vi "Teleop.vi"(10 "Match Info":T1={"Autonomous Elapsed Seconds"=0.0, "TeleOp Elapsed Seconds"=0.0, "Disabled Elapsed Seconds"=0.0, "Visited Autonomous"=FALSE, "Visited TeleOp"=FALSE, "Visited Disabled"=FALSE, "Autonomous Settings"={"Autonomous Style"=enum."Independent", "VI Refnum"=refnum}}, 11 "Call Context":T2) -> ()   [LabVIEW 2014]
doc: "This VI is called for each TeleOp packet received from the DS where the robot is not disabled. It is often used to read from the joysticks and update I/O or to update setpoints for timed control loops. It should complete and return within 20 milliseconds or it may miss DS packets."
uses:
  <vilib>/Rock Robotics/WPI/DriverStation/WPI_DriverStationDerivedRobotMode.ctl
  <vilib>/Rock Robotics/WPI/DriverStation/WPI_DriverStationMatch Info.ctl
  <vilib>/Rock Robotics/WPI/Joystick/WPI_JoystickGetSetRefNum.vi
  Robot Global Data.vi
  <vilib>/Rock Robotics/Network Tables/SD Write Boolean Array.vi
  <vilib>/Rock Robotics/Network Tables/SD Write Numeric Array.vi
  <vilib>/Rock Robotics/Network Tables/SD Read Boolean.vi
  <vilib>/Rock Robotics/Network Tables/SD Read Number.vi
  <vilib>/Rock Robotics/WPI/Compressor/WPI_CompressorGetSetRefNum.vi
panel:
  out "Wheel Lock":bool
  out "Closed Loop":bool
  out "Record":bool
  out "Sample Slider 0":dbl(slide) scale=0.0..5.0
  out "Sample Boolean 1":bool
  out "Sample Boolean 0":bool
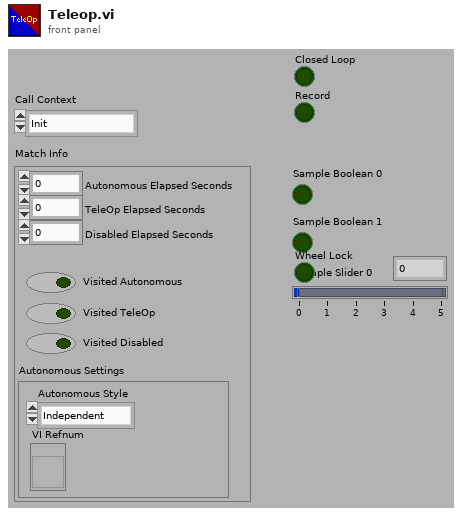
[diagram p1: front panel]
types:
  T1 = typedef "WPI_DriverStationMatch Info.ctl" = cluster{"Autonomous Elapsed Seconds":dbl, "TeleOp Elapsed Seconds":dbl, "Disabled Elapsed Seconds":dbl, "Visited Autonomous":bool, "Visited TeleOp":bool, "Visited Disabled":bool, "Autonomous Settings":cluster{"Autonomous Style":enum16{"Iterative", "Independent"}, "VI Refnum":refnum<vi>}}
  T2 = typedef "WPI_DriverStationDerivedRobotMode.ctl" = enum16{"Init", "Execute", "Stop"}
  T3 = typedef "WPI_JoystickDevRef.ctl" = cluster{"Device":T4}
  T4 = typedef "WPI_JoystickDeviceEnum.ctl" = enum16{"USB 0", "USB 1", "USB 2", "USB 3", "USB 4", "USB 5"}
  T5 = typedef "WPI_CompressorDevRef.ctl" = cluster{"DevStatus":errorcluster, "Pneumatics Control Module":u8}
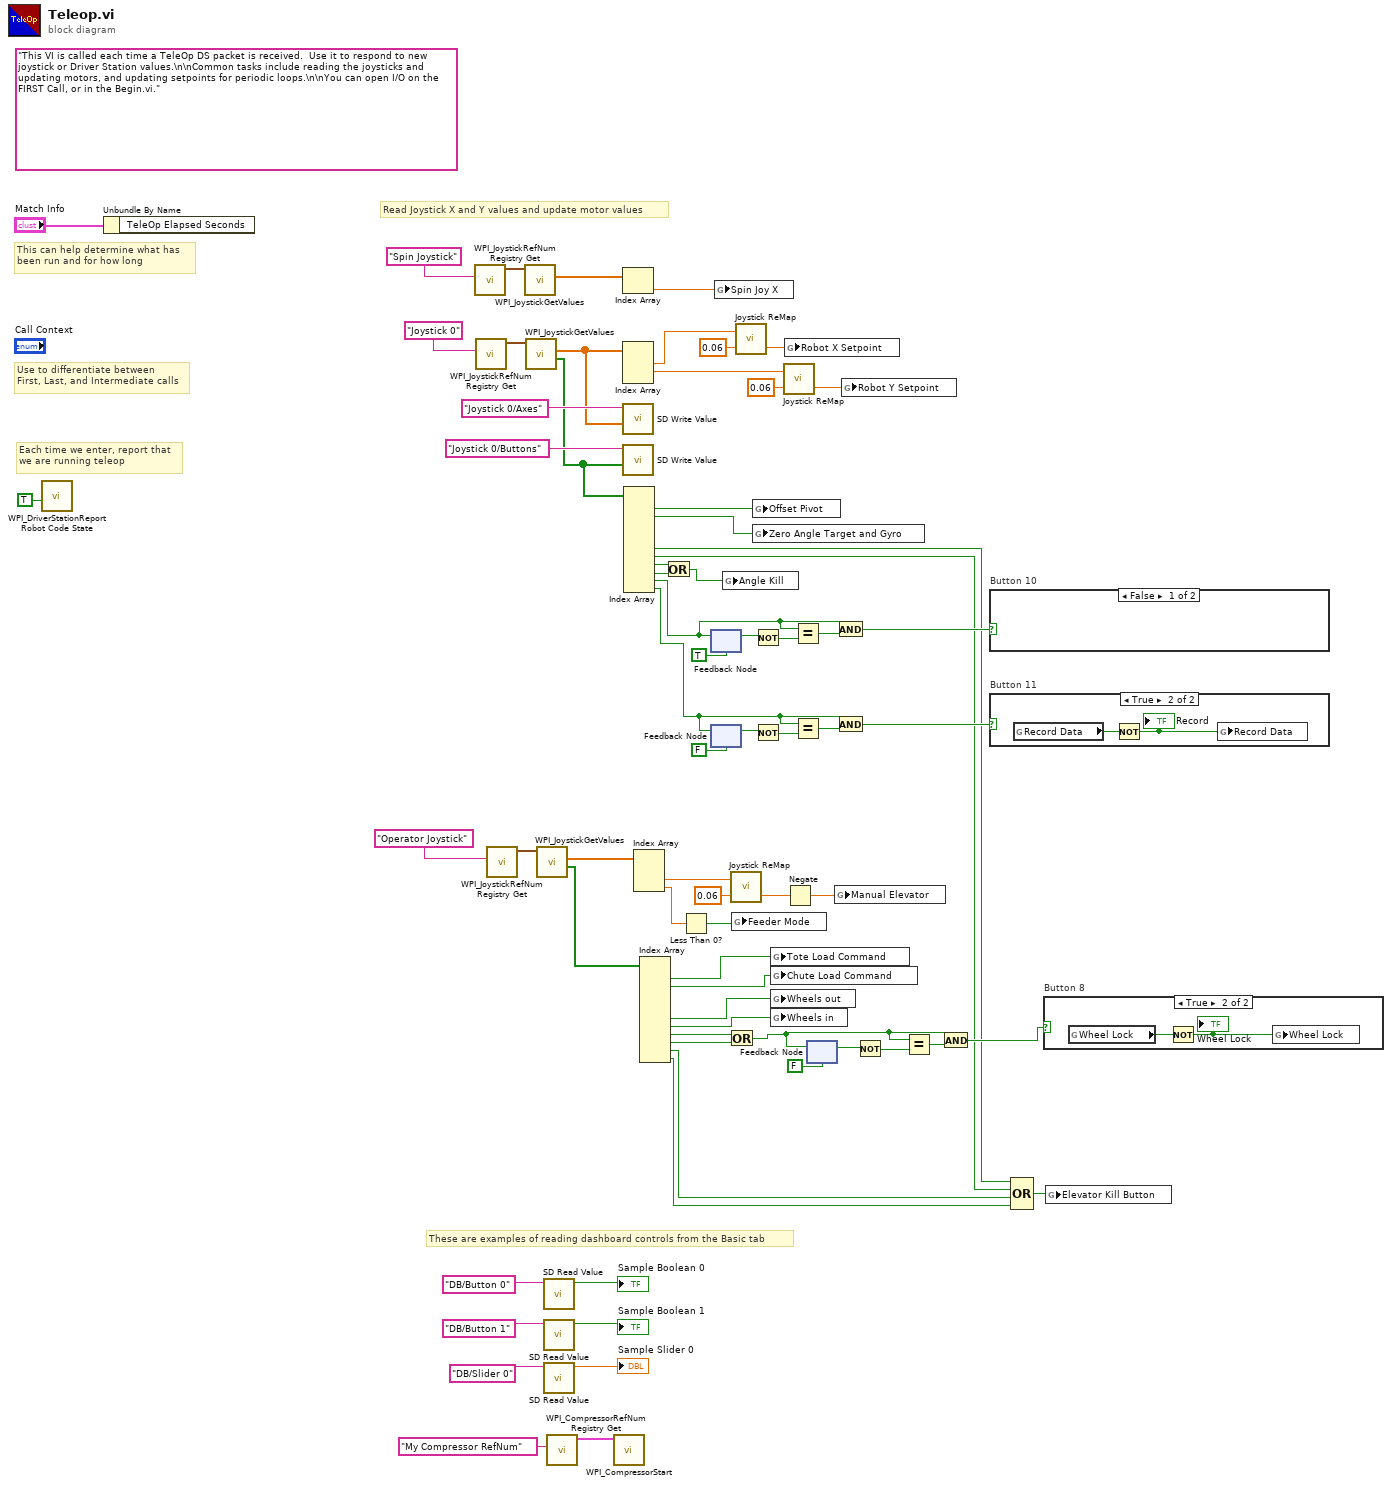
[diagram p0: block diagram]
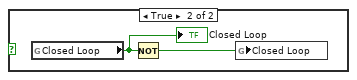
[diagram p3: hidden frame]
diagram:
  (unwired) "This VI is called each time a TeleOp DS packet is received.  Use it to respond to new joystick or Driver Station values.\n\nCommon tasks include reading the joysticks and updating motors, and updating setpoints for periodic loops.\n\nYou can open I/O on the FIRST Call, or in the Begin.vi."
  # "These are examples of reading dashboard controls from the Basic tab"
  # "Each time we enter, report that\nwe are running teleop"
  # "Use to differentiate between\nFirst, Last, and Intermediate calls"
  # "This can help determine what has\nbeen run and for how long"
  # "Read Joystick X and Y values and update motor values"
  n1 = call <vilib>:"WPI_DriverStationReport Robot Code State.vi"("TeleOp"=TRUE ("Autonomous")) -> ()  [unwired: 10 in, 1 out]
  n2 = Unbundle By Name("Match Info") -> ()  [unwired: 1 out]
  n3 = call <vilib>:"WPI_JoystickRefNum Registry Get.vi"("refnum name"="Spin Joystick") -> ("JoystickDevRef"=w40:T3)  [unwired: 1 in, 9 out]
  n4 = call <vilib>:"WPI_JoystickRefNum Registry Get.vi"("refnum name"="Joystick 0") -> ("JoystickDevRef"=w68:T3)  [unwired: 1 in, 9 out]
  n5 = call <vilib>:"WPI_JoystickRefNum Registry Get.vi"("refnum name"="Operator Joystick") -> ("JoystickDevRef"=w36:T3)  [unwired: 1 in, 9 out]
  n6 = call <vilib>:"WPI_JoystickGetValues.vi"("JoystickDevRef"=w40) -> ("Axes"=w38:dbl[])  [unwired: 6 in, 4 out]
  n7 = call <vilib>:"WPI_JoystickGetValues.vi"("JoystickDevRef"=w68) -> ("Buttons"=w57:bool[], "Axes"=w58:dbl[])  [unwired: 6 in, 3 out]
  n8 = call <vilib>:"WPI_JoystickGetValues.vi"("JoystickDevRef"=w36) -> ("Buttons"=w31:bool[], "Axes"=w37:dbl[])  [unwired: 6 in, 3 out]
  n9 = call-poly <vilib>:"SD Read Value.vi"("Name"="DB/Button 0" ("refnum name")) -> ("Boolean"=→"Sample Boolean 0":bool)  [unwired: 8 in, 2 out]
  n10 = call-poly <vilib>:"SD Read Value.vi"("Name"="DB/Button 1" ("refnum name")) -> ("Boolean"=→"Sample Boolean 1":bool)  [unwired: 8 in, 2 out]
  n11 = call-poly <vilib>:"SD Read Value.vi"("Name"="DB/Slider 0" ("refnum name")) -> ("Numeric"=→"Sample Slider 0":dbl)  [unwired: 8 in, 2 out]
  n12 = call <vilib>:"WPI_CompressorRefNum Registry Get.vi"("refnum name"="My Compressor RefNum") -> ("CompressorDevRef"=w50:T5)  [unwired: 9 in, 1 out]
  n13 = call <vilib>:"WPI_CompressorStart.vi"("CompressorDevRef"=w50) -> ()  [unwired: 9 in, 2 out]
  n14 = Index Array(array=w38) -> (element=w34:dbl)  [unwired: 1 in]
  n15 = Index Array(array=w58) -> (element #1=w42:dbl, element #2=w41:dbl)  [unwired: 3 in, 1 out]
  n16 = call-poly <vilib>:"SD Write Value.vi"("Numeric Array"=w58, "Name"="Joystick 0/Axes") -> ()  [unwired: 8 in, 2 out]
  n17 = call-poly <vilib>:"SD Write Value.vi"("Boolean Array"=w57, "Name"="Joystick 0/Buttons") -> ()  [unwired: 8 in, 2 out]
  n18 = Index Array(array=w57) -> (element #1=w23:bool, element #2=w12:bool, element #6=w6:bool, element #7=w5:bool, element #8=w3:bool, element #9=w2:bool, element #10=w43:bool, element #11=w52:bool)  [unwired: 11 in, 3 out]
  n19 = Index Array(array=w37) -> (element #2=w24:dbl, element #3=w28:dbl)  [unwired: 3 in, 1 out]
  n20 = Index Array(array=w31) -> (element #1=w11:bool, element #2=w10:bool, element #6=w22:bool, element #7=w21:bool, element #8=w9:bool, element #9=w8:bool, element #10=w30:bool, element #11=w29:bool)  [unwired: 11 in, 3 out]
  n21 = Or(x=w3, y=w2) -> (x .or. y?=w1:bool)
  n22 = Less Than 0?(x=w28) -> (x < 0?=w27:bool)
  n23 = feedback #1(TRUE) -> (w47:bool)
  n24 = feedback-in #1(w43) -> ()
  n25 = feedback-in #2(w52) -> ()
  n26 = feedback #2(FALSE) -> (w53:bool)
  n27 = global write "Robot Global Data.vi" "Spin Joy X"(w34) -> ()
  n28 = global write "Robot Global Data.vi" "Angle Kill"(w1) -> ()
  n29 = Or(x=w9, y=w8) -> (x .or. y?=w7:bool)
  n30 = call "Joystick ReMap.vi"("Deadband Size"=0.06, "Raw Value"=w24) -> ("Modified Value (x^2)"=w20:dbl)  [unwired: 1 out]
  n31 = global write "Robot Global Data.vi" "Feeder Mode"(w27) -> ()
  n32 = call "Joystick ReMap.vi"("Deadband Size"=0.06, "Raw Value"=w42) -> ("Modified Value (x^2)"=w19:dbl)  [unwired: 1 out]
  n33 = global write "Robot Global Data.vi" "Offset Pivot"(w23) -> ()
  n34 = global write "Robot Global Data.vi" "Zero Angle Target and Gyro"(w12) -> ()
  n35 = Not(x=w47) -> (.not. x?=w46:bool)
  n36 = Not(x=w53) -> (.not. x?=w54:bool)
  n37 = global write "Robot Global Data.vi" "Tote Load Command"(w11) -> ()
  n38 = global write "Robot Global Data.vi" "Chute Load Command"(w10) -> ()
  n39 = global write "Robot Global Data.vi" "Wheels out"(w22) -> ()
  n40 = global write "Robot Global Data.vi" "Wheels in"(w21) -> ()
  n41 = call "Joystick ReMap.vi"("Deadband Size"=0.06, "Raw Value"=w41) -> ("Modified Value (x^2)"=w18:dbl)  [unwired: 1 out]
  n42 = global write "Robot Global Data.vi" "Robot X Setpoint"(w19) -> ()
  n43 = Negate(x=w20) -> (-x=w25:dbl)
  n44 = Equal?(x=w43, y=w46) -> (x = y?=w45:bool)
  n45 = Equal?(x=w52, y=w54) -> (x = y?=w55:bool)
  n46 = feedback #3(FALSE) -> (w15:bool)
  n47 = feedback-in #3(w7) -> ()
  n48 = global write "Robot Global Data.vi" "Manual Elevator"(w25) -> ()
  n49 = And(x=w43, y=w45) -> (x .and. y?=w44:bool)
  n50 = And(x=w52, y=w55) -> (x .and. y?=w56:bool)
  n51 = global write "Robot Global Data.vi" "Robot Y Setpoint"(w18) -> ()
  n52 = Not(x=w15) -> (.not. x?=w16:bool)
  n53 = Equal?(x=w7, y=w16) -> (x = y?=w17:bool)
  n54 = And(x=w7, y=w17) -> (x .and. y?=w13:bool)
  n55 = case "Button 10" shown="False" w44 {
    frame False {
    }
    frame True {
      n56 = global read "Robot Global Data.vi" "Closed Loop"() -> (w71:bool)
      "Closed Loop" <- w71
      n57 = Not(x=w71) -> (.not. x?=w72:bool)
      n58 = global write "Robot Global Data.vi" "Closed Loop"(w72) -> ()
    }
  }
  n59 = case "Button 11" shown="True" w56 {
    frame False {
    }
    frame True {
      n60 = global read "Robot Global Data.vi" "Record Data"() -> (w74:bool)
      n61 = Not(x=w74) -> (.not. x?=w73:bool)
      "Record" <- w73
      n62 = global write "Robot Global Data.vi" "Record Data"(w73) -> ()
    }
  }
  n63 = Compound Arithmetic op=OR(w6, w5, w30, w29) -> (w4:bool)
  n64 = case "Button 8" shown="True" w13 {
    frame False {
    }
    frame True {
      n65 = global read "Robot Global Data.vi" "Wheel Lock"() -> (w76:bool)
      n66 = Not(x=w76) -> (.not. x?=w75:bool)
      "Wheel Lock" <- w75
      n67 = global write "Robot Global Data.vi" "Wheel Lock"(w75) -> ()
    }
  }
  n68 = global write "Robot Global Data.vi" "Elevator Kill Button"(w4) -> ()
